vi "Get MAC Info.vi"() -> ()   [LabVIEW 2013, in "ManagementClass.lvclass"]
uses:
  ManagementClass.lvclass
panel:
  out "元素":string
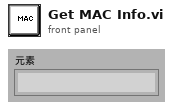
[diagram p1: front panel]
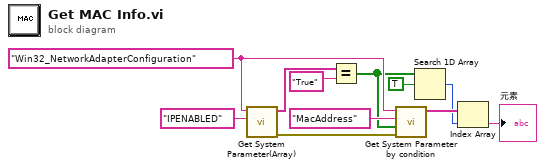
[diagram p0: block diagram]
diagram:
  w7 = "Win32_NetworkAdapterConfiguration" ("path")
  n1 = call "Get System Parameter(Array).vi"("propertyName"="IPENABLED", "path"=w7) -> ("error out"=w8:errorcluster, "Parameters"=w10:string[])  [unwired: 8 in]
  n2 = Equal?(x=w10, y="True") -> (x = y?=w5:bool[])
  n3 = call "Get System Parameter by condition.vi"("error in (no error)"=w8, "Enable"=w5, "propertyName"="MacAddress", "path"=w7) -> ("Parameters"=w3:string[])  [unwired: 6 in, 1 out]
  n4 = Search 1D Array(1D array=w5, element=TRUE ("元素")) -> (index of element=w2:i32)  [unwired: 1 in]
  n5 = Index Array(array=w3, index=w2) -> (element=→"元素":string)
